vi "IMG_PARAMS - GetTimeStamp.vi"(8 "error in (no error)":errorcluster, 11 "xiApi.NET.ImgParams":refnum<k24>) -> (0 "error out":errorcluster, 3 "xiApi.NET.ImgParams Out":refnum<k24>, 4 "TimeStamp":dbl)   [LabVIEW 2015]
doc: "Returns time stamp in seconds with microsecond precision."
uses:
  C:/GIT/Cameras3.x/Integrations/Labview/xiLib/xiLIB_32bit/xiLIB/xiCamLib/API/x86/xiApi.NET.dll
  xiLIB_32bit/xiLIB/xiCamLib/API/x86/xiApi.NET.dll
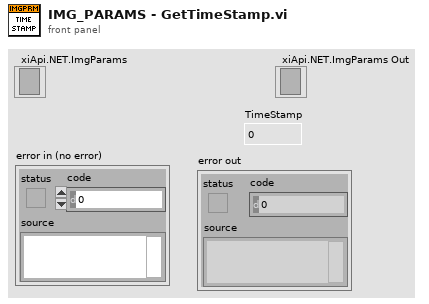
[diagram p1: front panel]
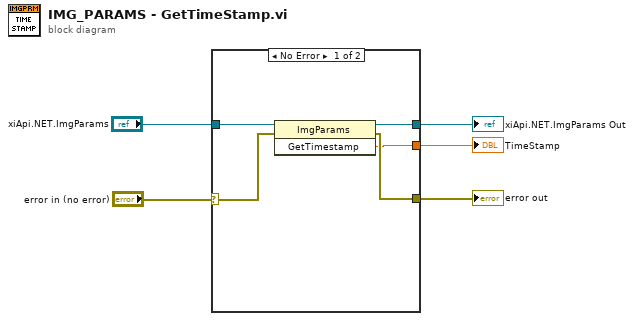
[diagram p0: block diagram]
diagram:
  n1 = case shown="No Error" "error in (no error)" {
    selector: "error in (no error)" -> [w8 w11]
    tunnel: "xiApi.NET.ImgParams" -> [w10 w12]
    tunnel: [w9 w12] -> w4
    tunnel: [w7 w11] -> w2
    tunnel: [w6 _] -> w1
    frame No Error {
      n2 = invoke class="ImgParams" method="GetTimestamp"(reference=w10, error in=w8) -> (reference out=w9:refnum<k24>, error out=w7:errorcluster, "GetTimestamp"=w6:dbl)  [unwired: 1 in]
    }
    frame Error {
    }
  }
  "xiApi.NET.ImgParams Out" <- w4
  "error out" <- w2
  "TimeStamp" <- w1
